vi "AssertsTrueorFalse.vi"(11 "error in (no error)":errorcluster) -> (15 "error out":errorcluster)   [LabVIEW 2016, in "DronaTest.lvlib"]
uses:
  APIs/Assert/AssertControlValue/False.vi
  <vilib>/addons/_JKI Toolkits/Caraya/classes/Assert/Assert Error.vi
  APIs/Assert/AssertControlValue/True.vi
  <vilib>/addons/_JKI Toolkits/Caraya/classes/Assert/Assert Not Error.vi
  DronaTest.lvlib
  <vilib>/addons/_JKI Toolkits/Caraya/classes/Test/Test.lvclass
  Drona.lvlib
  <vilib>/addons/_JKI Toolkits/Caraya/classes/Assert/Assert.lvclass
  APIs/Assert/AssertControlValue/AssertControlValue.lvlib
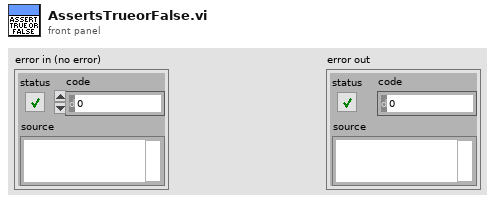
[diagram p1: front panel]
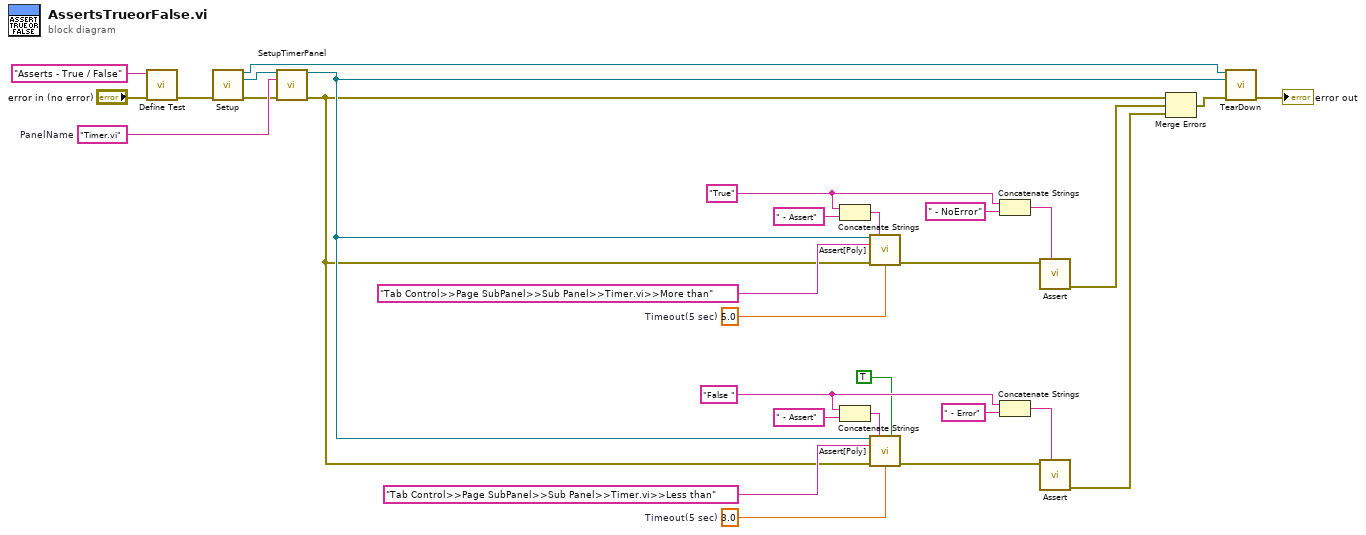
[diagram p0: block diagram]
diagram:
  w9 = "Timer.vi"  # PanelName
  w20 = 3.0  # Timeout(5 sec)
  w19 = "False " ("string")
  w21 = 5.0  # Timeout(5 sec)
  w22 = "True" ("string")
  n1 = call <vilib>:"Define Test.vi"("error in (no error)"="error in (no error)", "Label (VI Title)"="Asserts - True / False") -> ("error out"=w6:errorcluster)  [unwired: 9 in]
  n2 = call "Setup.vi"("error in (no error)"=w6) -> ("Application Ref"=w2:refnum<vi>, "VI out"=w7:refnum<vi>, "error out"=w8:errorcluster)  [unwired: 12 in]
  n3 = call "SetupTimerPanel.vi"("VI in"=w7, "Panel Name"=w9, "error in (no error)"=w8) -> ("VI out"=w5:refnum<vi>, "error out"=w1:errorcluster)  [unwired: 11 in]
  n4 = Concatenate Strings(w22, " - Assert" ("string")) -> (w24:string)
  n5 = Concatenate Strings(w19, " - Assert" ("string")) -> (w17:string)
  n6 = call-poly "Assert[Poly].vi"("VI Reference In"=w5, "Test Label"=w24, "Control Path"="Tab Control>>Page SubPanel>>Sub Panel>>Timer.vi>>More than", "Error In"=w1, "Timeout(5 sec)"=w21) -> ("Error Out"=w25:errorcluster)  [unwired: 9 in, 1 out]
  n7 = call-poly "Assert[Poly].vi"("VI Reference In"=w5, "Test Label"=w17, "Assert Only? (F)"=TRUE, "Control Path"="Tab Control>>Page SubPanel>>Sub Panel>>Timer.vi>>Less than", "Error In"=w1, "Timeout(5 sec)"=w20) -> ("Error Out"=w16:errorcluster)  [unwired: 8 in, 1 out]
  n8 = Concatenate Strings(w22, " - NoError" ("string")) -> (w23:string)
  n9 = Concatenate Strings(w19, " - Error" ("string")) -> (w18:string)
  n10 = call-poly <vilib>:"Assert.vi"("Label"=w23, "Not Error?"=w25) -> ("error out"=w11:errorcluster)  [unwired: 9 in]
  n11 = call-poly <vilib>:"Assert.vi"("Label"=w18, "Error?"=w16) -> ("error out"=w10:errorcluster)  [unwired: 9 in]
  n12 = Merge Errors(w1, w11, w10) -> (w4:errorcluster)
  n13 = call "TearDown.vi"("Application Ref"=w2, "VI in"=w5, "error in (no error)"=w4) -> ("error out"=→"error out":errorcluster)  [unwired: 12 in]
